vi "ReleaseSensorQueue.vi"(8 "error in (no error)":errorcluster, 11 "AnalysisPluginsBase In":refnum<class "AnalysisPluginsBase.lvclass">) -> (0 "error out":errorcluster, 3 "AnalysisPluginsBase Out":refnum<class "AnalysisPluginsBase.lvclass">)   [LabVIEW 2018, in "AnalysisPlugins.lvlib" / "AnalysisPluginsBase.lvclass"]
uses:
  AnalysisPluginsBase.lvclass
  Typedefs/SensorQueue.ctl
  Typedefs/clSensorData.ctl
  AnalysisPluginsBase.lvclass/AnalysisPluginsBase.ctl
  Accessors/Read SensorQue.vi
  Accessors/Write SensorQue.vi
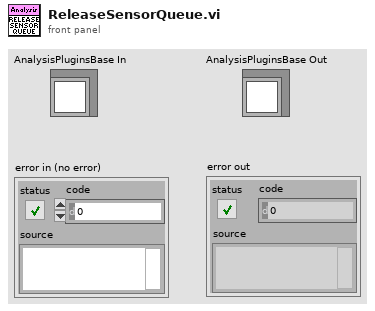
[diagram p1: front panel]
types:
  T1 = typedef "SensorQueue.ctl" = refnum<queue>
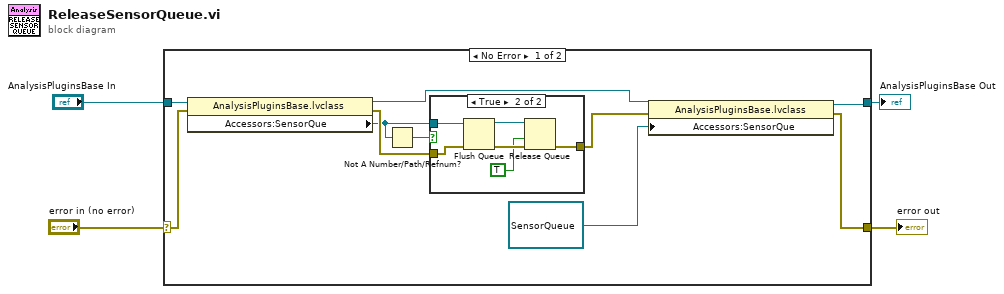
[diagram p0: block diagram]
diagram:
  n1 = case shown="No Error" "error in (no error)" {
    selector: "error in (no error)" -> [w13 w22]
    tunnel: "AnalysisPluginsBase In" -> [w14 w23]
    tunnel: [w6 w23] -> w2
    tunnel: [w5 w22] -> w1
    frame No Error {
      n2 = property class="AnalysisPluginsBase.lvclass"(reference=w14, error in=w13) -> (reference out=w9:refnum<class "AnalysisPluginsBase.lvclass">, error out=w11:errorcluster, "Accessors:SensorQue"=w10:T1)
      n3 = Not A Number/Path/Refnum?(number/path/refnum=w10) -> (NaN/Path/Refnum?=w12:bool)
      n4 = case shown="True" w12 {
        tunnel: w11 -> [w15 w20]
        tunnel: w10 -> [_ w21]
        tunnel: [w15 w16] -> w7
        frame False {
        }
        frame True {
          n5 = Flush Queue(queue=w21, error in (no error)=w20) -> (queue out=w18:T1, error out=w19:errorcluster)  [unwired: 1 out]
          n6 = Release Queue(queue=w18, force destroy? (F)=TRUE, error in (no error)=w19) -> (error out=w16:errorcluster)  [unwired: 2 out]
        }
      }
      n7 = property class="AnalysisPluginsBase.lvclass"(reference=w9, error in=w7, "Accessors:SensorQue"=T1 refnum ("SensorQue")) -> (reference out=w6:refnum<class "AnalysisPluginsBase.lvclass">, error out=w5:errorcluster)
    }
    frame Error {
    }
  }
  "AnalysisPluginsBase Out" <- w2
  "error out" <- w1
